vi "Edit Shared Resource.vi"(8 "error in (no error)":errorcluster, 10 "RID":string, 11 "Controller in":refnum<class "Controller.lvclass">) -> (0 "error out":errorcluster, 3 "Controller out":refnum<class "Controller.lvclass">)   [LabVIEW 2013, in "SET Project Editor.lvlib" / "Controller.lvclass"]
uses:
  Controller.lvclass
  Controller.lvclass/Controller.ctl
  SET Project Data/Project Data Class/Project Data.lvclass
  <vilib>/ActorFramework/Message Enqueuer/Message Enqueuer.lvclass/Message Enqueuer.ctl
  <vilib>/ActorFramework/Message Enqueuer/Enqueue.vi
  <vilib>/ActorFramework/Message Priority Queue/Priority Enqueue.vi
  SET Project Data/Resource Data Class/Resource Data.lvclass
  UI View Messages/UI Refresh Data Msg/UI Refresh Data Msg.lvclass
  SET Project Editor.lvlib
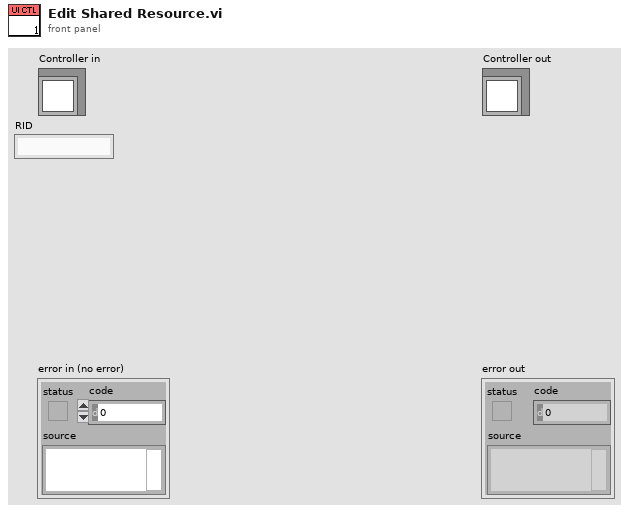
[diagram p1: front panel]
types:
  T1 = typedef "SET Project Data.lvlib/ProjFile_Resource Entry.ctl" = cluster{"RID":string, "Tag":string, "Strings [] (UTF-16)":string[], "Shared?":bool}
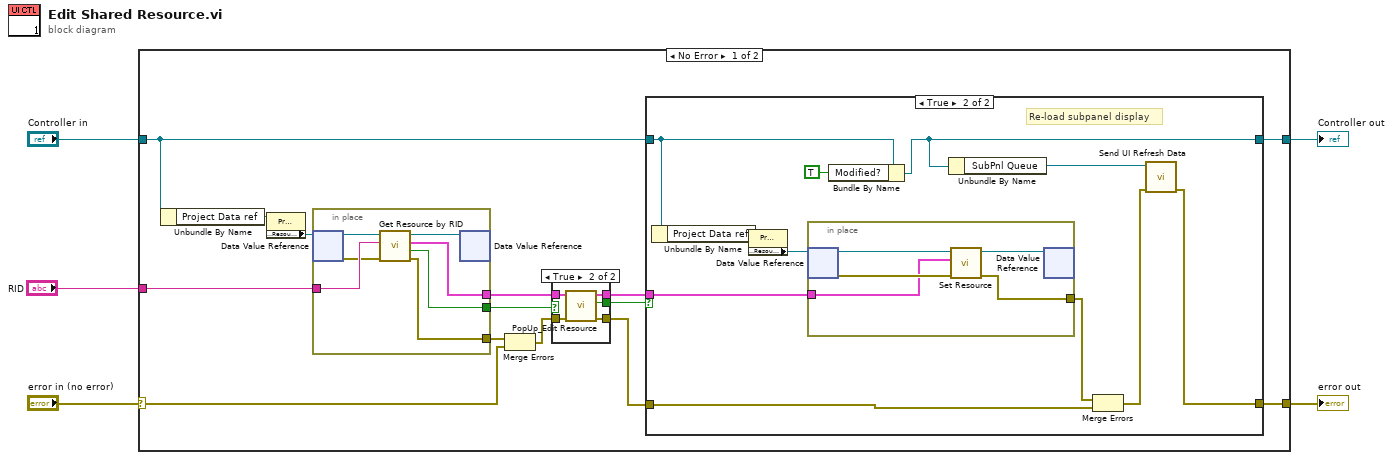
[diagram p0: block diagram]
diagram:
  n1 = case shown="No Error" "error in (no error)" {
    selector: "error in (no error)" -> [w10 w53]
    tunnel: [w16 w53] -> w4
    tunnel: [w18 w52] -> w2
    tunnel: "Controller in" -> [w14 w52]
    tunnel: "RID" -> [w12 _]
    frame No Error {
      n2 = Unbundle By Name(w14) -> ("Project Data ref"=w15:refnum<data-value>)
      n3 = property class="Project Data.lvclass"(reference=w15) -> ("Properties:Resource Data ref"=w13:refnum<data-value>)  [unwired: 1 in, 2 out]
      n4 = in-place {
        in-place-border: w12 -> [w31]
        in-place-border: [w29] -> w6
        in-place-border: [w28] -> w8
        in-place-border: [w27] -> w11
        n5 = in-place-dvr #1(w13) -> (w33:refnum<class "Resource Data.lvclass">, w30:errorcluster)
        n6 = call "Get Resource by RID.vi"("error in (no error)"=w30, "RID"=w31, "LangFile in"=w33) -> ("error out"=w27:errorcluster, "Found?"=w29:bool, "Resource"=w28:T1, "LangFile out"=w32:refnum<class "Resource Data.lvclass">)  [unwired: 4 in, 1 out]
        n7 = in-place-dvr #1(w32) -> ()  [unwired: 2 out]
      }
      n8 = Merge Errors(w11, w10) -> (w9:errorcluster)
      n9 = case shown="True" w6 {
        tunnel: [w21 w26] -> w19
        tunnel: [w20 w25] -> w17
        tunnel: w9 -> [w20 w24]
        tunnel: w8 -> [w21 w23]
        tunnel: [_ w22] -> w7
        frame False {
        }
        frame True {
          n10 = call "PopUp_Edit Resource.vi"("error in (no error)"=w24, "Resource in"=w23) -> ("error out"=w25:errorcluster, "OK Pressed?"=w22:bool, "Resource out"=w26:T1)  [unwired: 7 in]
        }
      }
      n11 = case shown="True" w7 {
        tunnel: w19 -> [_ w43]
        tunnel: w14 -> [w35 w42]
        tunnel: [w35 w39] -> w18
        tunnel: w17 -> [w34 w40]
        tunnel: [w34 w36] -> w16
        frame False {
        }
        frame True {
          # "Re-load subpanel display"
          n12 = Unbundle By Name(w42) -> ("Project Data ref"=w46:refnum<data-value>)
          n13 = property class="Project Data.lvclass"(reference=w46) -> ("Properties:Resource Data ref"=w45:refnum<data-value>)  [unwired: 1 in, 2 out]
          n14 = in-place {
            in-place-border: w43 -> [w47]
            in-place-border: [w48] -> w41
            n15 = in-place-dvr #2(w45) -> (w51:refnum<class "Resource Data.lvclass">, w49:errorcluster)
            n16 = call "Set Resource.vi"("error in (no error)"=w49, "Resource"=w47, "LangFile in"=w51) -> ("error out"=w48:errorcluster, "LangFile out"=w50:refnum<class "Resource Data.lvclass">)  [unwired: 7 in]
            n17 = in-place-dvr #2(w50) -> ()  [unwired: 2 out]
          }
          n18 = Bundle By Name(cluster=w42, "Modified?"=TRUE) -> (w39:refnum<class "Controller.lvclass">)
          n19 = Unbundle By Name(w39) -> ("SubPnl Queue"=w38:refnum<class "Message Enqueuer.lvclass">)
          n20 = Merge Errors(w41, w40) -> (w37:errorcluster)
          n21 = call "Send UI Refresh Data.vi"("error in (no error)"=w37, "Message Enqueuer"=w38) -> ("error out"=w36:errorcluster)  [unwired: 8 in, 1 out]
        }
      }
    }
    frame Error {
    }
  }
  "error out" <- w4
  "Controller out" <- w2
